vi "RW Match ROI.vi"(7 "Read/Write":enum16{"Read", "Write"}(ring), 8 "error in (no error)":errorcluster, 11 "Inspec part":T1) -> (0 "error out":errorcluster)   [LabVIEW 2017]
uses:
  File/File.lvlib
  File/Control/Parent path.ctl
  <vilib>/Utility/config.llb/NI_LVConfig.lvlib
  <vilib>/Utility/config.llb/Read Key (Double).vi
  Section and key name.vi
  <vilib>/Utility/config.llb/Read Key (I32).vi
  Toolbox/Toolbox.lvlib
  Toolbox/Control/CVT Action.ctl
  <vilib>/Utility/config.llb/Write Key (I32).vi
  <vilib>/Utility/config.llb/Write Key (Double).vi
  Toolbox/Control/CVT name.vi
  Use Module/Algorithm Loop/Gentex Algo/inspec part.ctl
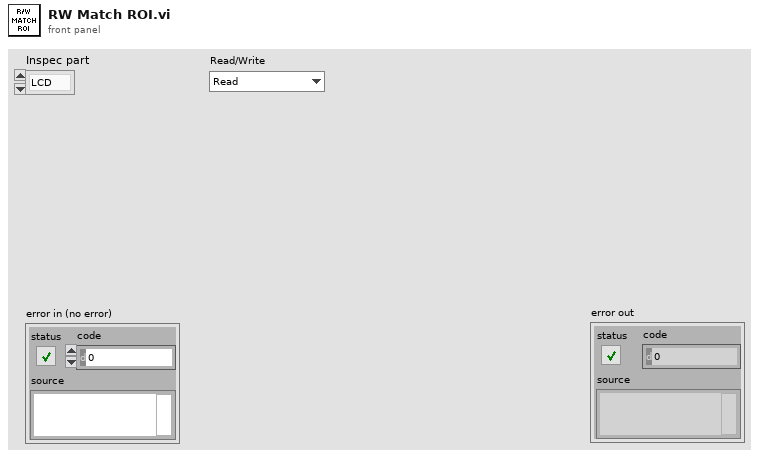
[diagram p1: front panel]
types:
  T1 = typedef "Algorithm API.lvlib/inspec part.ctl" = enum16{"LCD", "Housing"}
  T2 = typedef "Toolbox.lvlib/CVT Action.ctl" = enum16{"Set", "Replace", "Get", "Check", "Delete", "Delete All"}
  T3 = typedef "ROI Descriptor" = cluster{"Global Rectangle":i32[], "Contours":cluster{"ID":enum32{"External", "Internal"}, "Type":u32, "Coordinates":i32[]}[]}
  T4 = typedef "File.lvlib/Parent path.ctl" = enum16{"Project", "Setting", "Log"}
  T5 = typedef "IMAQ Rectangle" = cluster{"Left":i32, "Top":i32, "Right":i32, "Bottom":i32, "Rotation":dbl}
  T6 = typedef "NI_LVConfig.lvlib/Config Data RefNum.ctl" = refnum<k1>
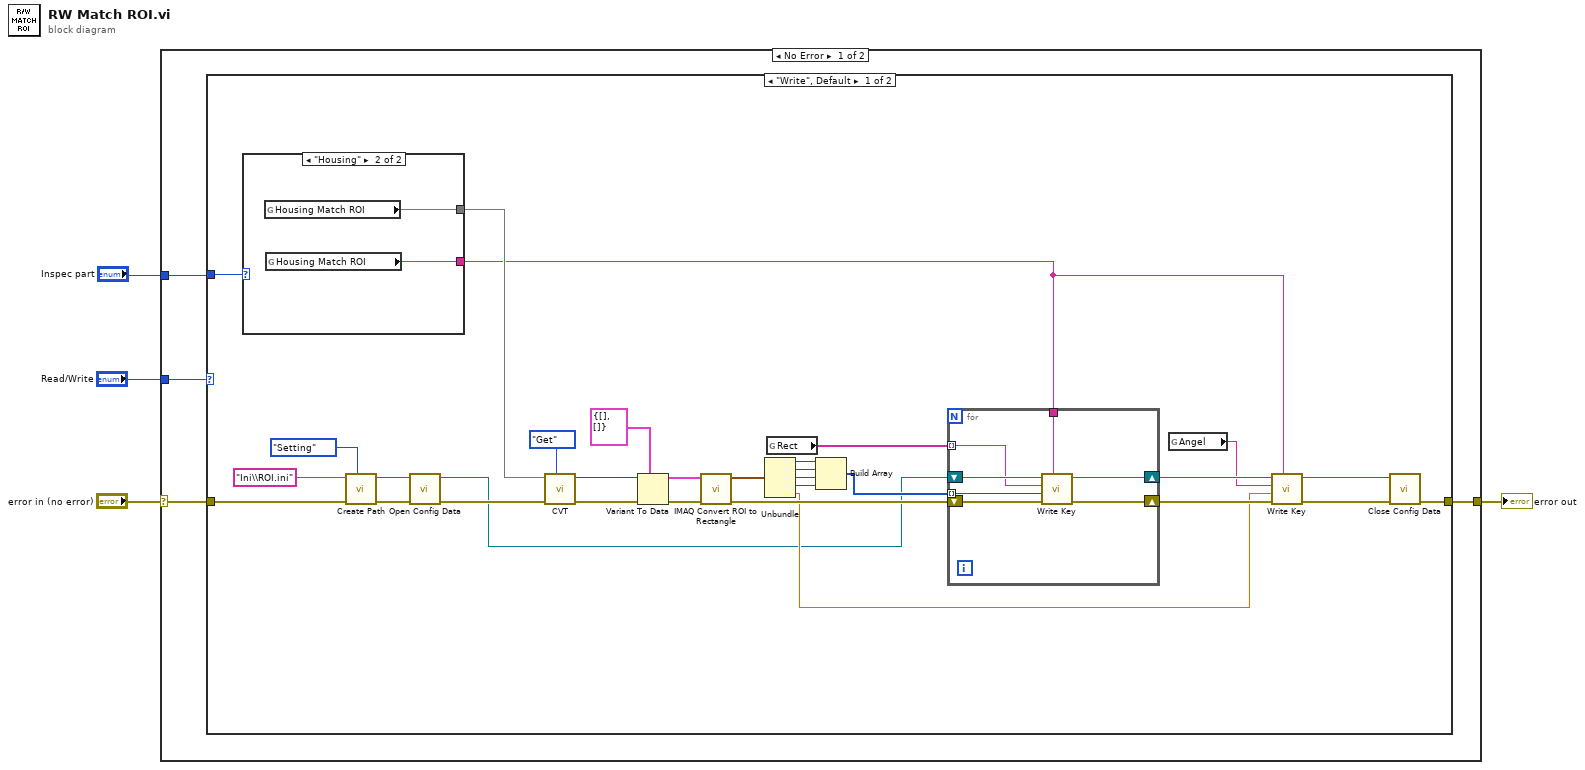
[diagram p0: block diagram]
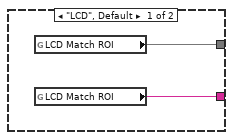
[diagram p2: hidden frame]
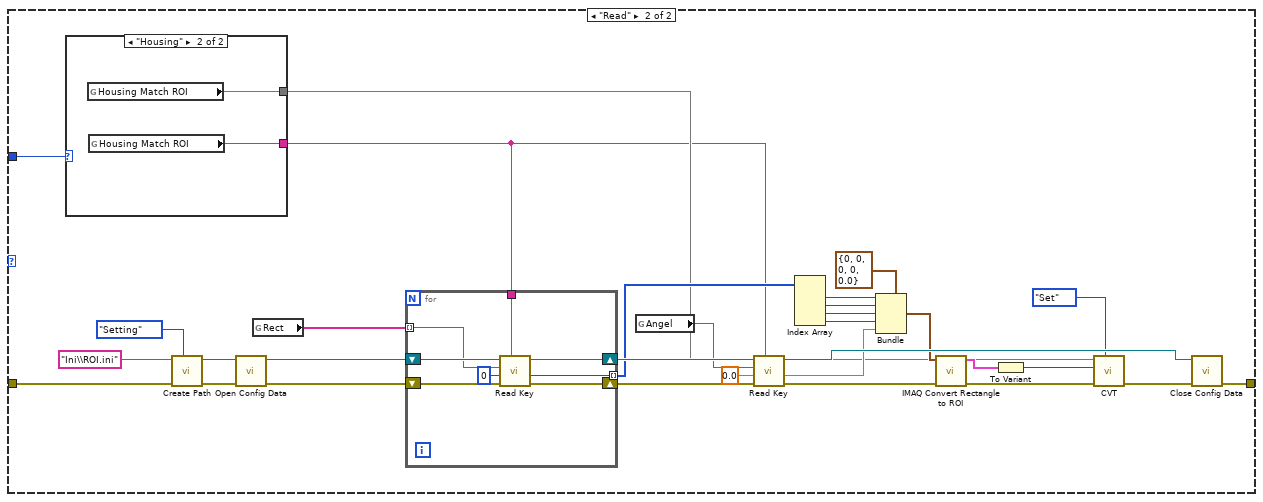
[diagram p3: hidden frame]
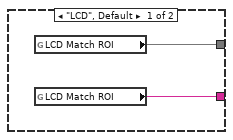
[diagram p4: hidden frame]
diagram:
  n1 = case shown="No Error" "error in (no error)" {
    selector: "error in (no error)" -> [w8 w94]
    tunnel: [w7 w94] -> w3
    tunnel: "Read/Write" -> [w6 _]
    tunnel: "Inspec part" -> [w5 _]
    frame No Error {
      n2 = case shown="\"Write\", Default" w6 {
        tunnel: w8 -> [w39 w81]
        tunnel: [w33 w74] -> w7
        tunnel: w5 -> [w11 w53]
        frame "Write", Default {
          n3 = case shown="\"Housing\"" w11 {
            tunnel: [w41 w42] -> w9
            tunnel: [w40 w43] -> w10
            frame "LCD", Default {
              n4 = global read "CVT name.vi" "LCD Match ROI"() -> (w40)
              n5 = global read "Section and key name.vi" "LCD Match ROI"() -> (w41:string)
            }
            frame "Housing" {
              n6 = global read "CVT name.vi" "Housing Match ROI"() -> (w43)
              n7 = global read "Section and key name.vi" "Housing Match ROI"() -> (w42:string)
            }
          }
          n8 = call "Create Path.vi"("Parent path"=Parent_path."Setting", "error in (no error)"=w39, "Directory"="Ini\\ROI.ini") -> ("error out"=w37:errorcluster, "Path"=w36:path)  [unwired: 7 in]
          n9 = call <vilib>:"Open Config Data.vi"("error in (no error)"=w37, "configuration file path"=w36) -> ("error out"=w35:errorcluster, "refnum"=w13:T6)  [unwired: 7 in, 1 out]
          n10 = call "CVT.vi"("Action"=CVT_Action."Get", "error in (no error)"=w35, "Key"=w10) -> ("error out"=w27:errorcluster, "Value out"=w25:variant)  [unwired: 6 in, 1 out]
          n11 = Variant To Data(error in=w27, type=T3 {"Global Rectangle"=[], "Contours"=[]} ("ROI Descriptor"), Variant=w25) -> (data=w21:T3, error out=w26:errorcluster)
          n12 = call "IMAQ Convert ROI to Rectangle"("error in (no error)"=w26, "ROI Descriptor"=w21) -> ("error out"=w22:errorcluster, "Rectangle"=w20:T5)  [unwired: 7 in]
          n13 = Unbundle(w20) -> ("Left"=w18:i32, "Top"=w17:i32, "Right"=w16:i32, "Bottom"=w15:i32, "Rotation"=w19:dbl)
          n14 = global read "Section and key name.vi" "Rect"() -> (w29:string[])
          n15 = Build Array(w18, w17, w16, w15) -> (w14:i32[])
          n16 = for {
            shift-right: [w48] -> w31
            shift-left: w13 -> [w50]
            shift-right: [w47] -> w30
            shift-left: w22 -> [w49]
            tunnel: w29 -> [w46] mode=indexing
            tunnel: w9 -> [w45]
            tunnel: w14 -> [w44] mode=indexing
            n17 = call-poly <vilib>:"Write Key.vi"("section"=w45, "error in (no error)"=w49, "value"=w44, "key"=w46, "refnum"=w50) -> ("error out"=w47:errorcluster, "refnum out"=w48:T6)  [unwired: 4 in, 1 out]
          }
          n18 = global read "Section and key name.vi" "Angel"() -> (w28:string)
          n19 = call-poly <vilib>:"Write Key.vi"("section"=w9, "error in (no error)"=w30, "value"=w19, "key"=w28, "refnum"=w31) -> ("error out"=w34:errorcluster, "refnum out"=w32:T6)  [unwired: 4 in, 1 out]
          n20 = call <vilib>:"Close Config Data.vi"("error in (no error)"=w34, "refnum"=w32) -> ("error out"=w33:errorcluster)  [unwired: 8 in, 1 out]
        }
        frame "Read" {
          n21 = case shown="\"Housing\"" w53 {
            tunnel: [w83 w84] -> w51
            tunnel: [w82 w85] -> w52
            frame "LCD", Default {
              n22 = global read "CVT name.vi" "LCD Match ROI"() -> (w82)
              n23 = global read "Section and key name.vi" "LCD Match ROI"() -> (w83:string)
            }
            frame "Housing" {
              n24 = global read "CVT name.vi" "Housing Match ROI"() -> (w85)
              n25 = global read "Section and key name.vi" "Housing Match ROI"() -> (w84:string)
            }
          }
          n26 = call "Create Path.vi"("Parent path"=Parent_path."Setting", "error in (no error)"=w81, "Directory"="Ini\\ROI.ini") -> ("error out"=w79:errorcluster, "Path"=w78:path)  [unwired: 7 in]
          n27 = call <vilib>:"Open Config Data.vi"("error in (no error)"=w79, "configuration file path"=w78) -> ("error out"=w76:errorcluster, "refnum"=w77:T6)  [unwired: 7 in, 1 out]
          n28 = global read "Section and key name.vi" "Rect"() -> (w70:string[])
          n29 = for {
            shift-right: [w91] -> w72
            shift-left: w77 -> [w93]
            shift-right: [w90] -> w71
            shift-left: w76 -> [w92]
            tunnel: [w89] -> w67 mode=indexing
            tunnel: w70 -> [w88] mode=indexing
            tunnel: w51 -> [w87]
            n30 = call-poly <vilib>:"Read Key.vi"("section"=w87, "error in (no error)"=w92, "default value"=0, "key"=w88, "refnum"=w93) -> ("error out"=w90:errorcluster, "value"=w89:i32, "refnum out"=w91:T6)  [unwired: 3 in, 1 out]
          }
          n31 = global read "Section and key name.vi" "Angel"() -> (w69:string)
          n32 = call-poly <vilib>:"Read Key.vi"("section"=w51, "error in (no error)"=w71, "default value"=0.0, "key"=w69, "refnum"=w72) -> ("error out"=w68:errorcluster, "value"=w61:dbl, "refnum out"=w73:T6)  [unwired: 3 in, 1 out]
          n33 = Index Array(array=w67) -> (element #1=w65:i32, element #2=w64:i32, element #3=w63:i32, element #4=w62:i32)  [unwired: 4 in]
          n34 = Bundle(cluster=T5 {"Left"=0, "Top"=0, "Right"=0, "Bottom"=0, "Rotation"=0.0} ("Rectangle"), "Left"=w65, "Top"=w64, "Right"=w63, "Bottom"=w62, "Rotation"=w61) -> (w60:T5)
          n35 = call "IMAQ Convert Rectangle to ROI"("error in (no error)"=w68, "Rectangle"=w60) -> ("error out"=w59:errorcluster, "ROI Descriptor"=w58:T3)  [unwired: 7 in]
          n36 = To Variant(anything=w58) -> (Variant=w57:variant)
          n37 = call "CVT.vi"("Action"=CVT_Action."Set", "error in (no error)"=w59, "Value in"=w57, "Key"=w52) -> ("error out"=w75:errorcluster)  [unwired: 5 in, 2 out]
          n38 = call <vilib>:"Close Config Data.vi"("error in (no error)"=w75, "refnum"=w73) -> ("error out"=w74:errorcluster)  [unwired: 8 in, 1 out]
        }
      }
    }
    frame Error {
    }
  }
  "error out" <- w3
